vi "Мажор_не_работает_дтектор.vi"() -> ()   [LabVIEW 2017]
panel:
  out "s? t:f":dbl
  out "element":dbl
  out "После ошибки":dbl[](array[numeric])
  out "2-х массив на выходе 3":dbl[][](array[numeric])
  in  "Размер окна":i32=4
  out "см. 1.5":dbl[][](array[numeric])
  out "Декодированное сообщение":dbl[](array[numeric])
  out "Детектированное сообщение":dbl[](array[numeric])
  out "До ошибки":dbl[](array[numeric])
  in  "Кол-во копий":i32=5
  out "Массиве":dbl[](array[numeric])
  in  "Кол-во элементов":i32=16
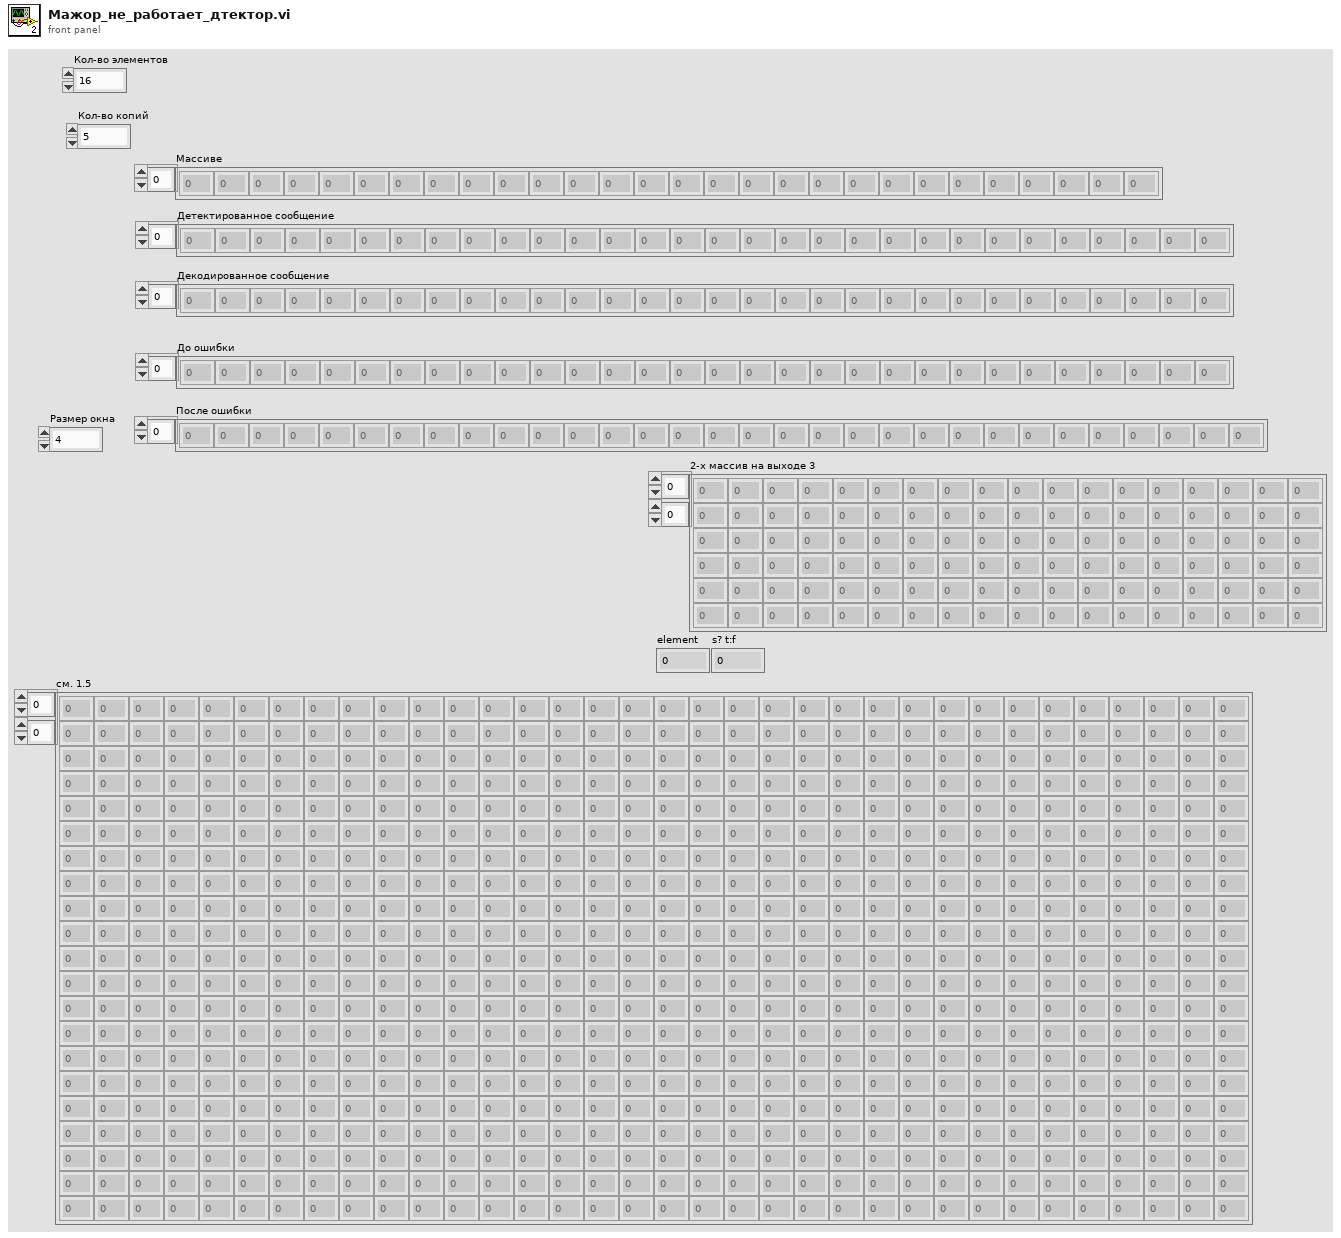
[diagram p1: front panel]
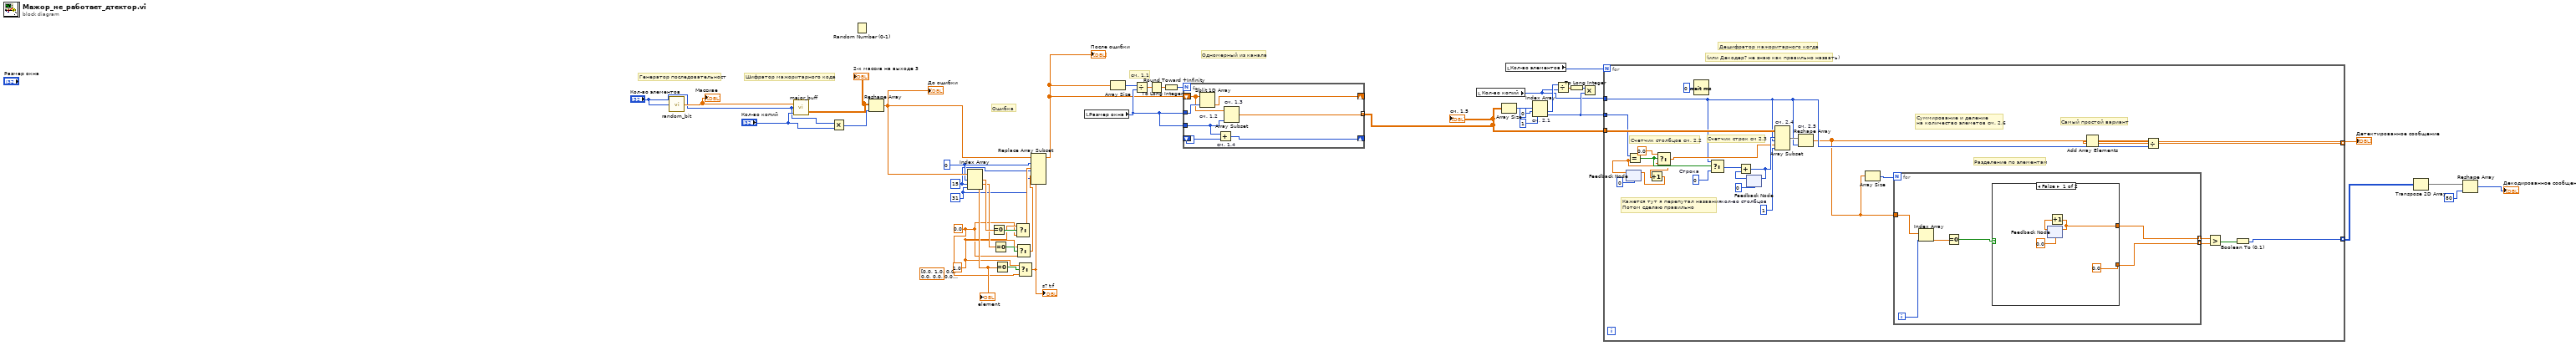
[diagram p0: block diagram]
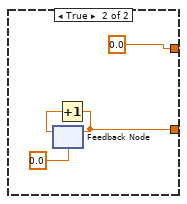
[diagram p2: hidden frame]
diagram:
  (unwired) dbl[] [0.0, 1.0, 0.0, 0.0, 0.0, 0.0, 0.0, 1.0, 1.0, 1.0, 0.0, 1.0, 1.0, 0.0, 0.0, 1.0] ("Декодированное сообщение")
  w12 = 1.0
  w11 = 0.0
  w5 = 31
  w6 = 15
  w7 = 0
  # "Ошибка"
  # "Одномерный из канала"
  # "см. 1.1"
  # "(или Декодер? не знаю как правильно назвать)"
  # "Дешифратор мажоритарного когда"
  # "Шифратор мажоритарного кода"
  # "Генератор последовательност"
  n1 = call "random_bit.vi"("Количество бит"="Кол-во элементов") -> ("Биты на выходе 1"=w41:dbl[])
  "Массиве" <- w41
  n2 = call "major_buff.vi"("Кол-во копий"="Кол-во копий", "Размер окна"="Кол-во элементов", "Биты на выходе 1"=w41) -> ("Подготовленный к отправке мажоритарный код"=w21:dbl[][])  [unwired: 1 out]
  "2-х массив на выходе 3" <- w21
  n3 = Multiply(x="Кол-во элементов", y="Кол-во копий") -> (x*y=w40:i32)
  n4 = Random Number (0-1)() -> ()  [unwired: 1 out]
  n5 = Reshape Array(w21, w40) -> (w19:dbl[])
  "До ошибки" <- w19
  n6 = Index Array(array=w19, index #1=w7, index #2=w6, index #3=w5) -> (element #1=w18:dbl, element #2=w17:dbl, element #3=w16:dbl)
  "element" <- w16
  n7 = Equal To 0?(x=w18) -> (x = 0?=w15:bool)
  n8 = Equal To 0?(x=w17) -> (x = 0?=w14:bool)
  n9 = Equal To 0?(x=w16) -> (x = 0?=w13:bool)
  n10 = Select(t=w12, s=w15, f=w11) -> (s? t:f=w10:dbl)
  n11 = Select(t=w12, s=w14, f=w11) -> (s? t:f=w9:dbl)
  n12 = Select(t=w12, s=w13, f=w11) -> (s? t:f=w8:dbl)
  "s? t:f" <- w8
  n13 = Replace Array Subset(array=w19, new element #1=w10, index #1=w7, new element #2=w9, index #2=w6, new element #3=w8, index #3=w5) -> (w24:dbl[])
  "После ошибки" <- w24
  n14 = local read "Размер окна"() -> (w31:i32)
  n15 = Array Size(array=w24) -> (size(s)=w30:i32)
  n16 = Divide(x=w30, y=w31) -> (x/y=w29:dbl)
  n17 = Round Toward +Infinity(x=w29) -> (ceil(x): smallest int >= x=w28:dbl)
  n18 = To Long Integer(number=w28) -> (32bit integer=w27:i32)
  n19 = for {
    N: w27 -> [_]
    shift-right: [w48] -> _
    shift-left: w24 -> [w46]
    tunnel: w31 -> [w47]
    shift-right: [w44] -> _
    shift-left: _ -> [w43]
    tunnel: w31 -> [w45]
    tunnel: [w42] -> w20 mode=indexing
    n20 = Split 1D Array "см. 1.2"(array=w46, index=w47) -> (second subarray=w48:dbl[])  [unwired: 1 out]
    n21 = Add "см. 1.4"(x=w45, y=w43) -> (x+y=w44:i32)
    n22 = Array Subset "см. 1.3"(array=w46, length=w45) -> (w42:dbl[])  [unwired: 1 in]
  }
  "см. 1.5" <- w20
  n23 = local read "Кол-во копий"() -> (w32:i32)
  n24 = Array Size(array=w20) -> (size(s)=w39:i32[])
  n25 = local read "Кол-во элементов"() -> (w25:i32)
  n26 = Index Array "см. 2.1"(array=w39, index #1=0 ("index"), index #2=1 ("index")) -> (element #1=w36:i32, element #2=w35:i32)
  n27 = Divide(x=w36, y=w32) -> (x/y=w34:dbl)
  n28 = To Long Integer(number=w34) -> (32bit integer=w33:i32)
  n29 = Multiply(x=w33, y=w35) -> ()  [unwired: 1 out]
  n30 = for {
    N: w25 -> [_]
    tunnel: w20 -> [w72]
    tunnel: w35 -> [w64]
    tunnel: w32 -> [w56]
    tunnel: [w55] -> w26 mode=indexing
    tunnel: [w49] -> w4 mode=indexing
    w71 = 1  # кол-во столбцов
    w62 = 0  # Строка
    # "Разделение по элементам"
    # "Самый простой вариант"
    # "Суммирование и деление \nна количество элеметов см. 2.6"
    # "Кажется тут я перепутал названия  \nПотом сделаю правильно"
    # "Счетчик строк см 2.3"
    # "Счетчик столбцов см. 2.2"
    n31 = feedback #1(0) -> (w60:dbl)
    n32 = Equal?(x=w64, y=w60) -> (x = y?=w66:bool)
    n33 = Select(t=0.0, s=w66, f=w60) -> (s? t:f=w59:dbl)
    n34 = Increment(x=w59) -> (x+1=w58:dbl)
    n35 = feedback-in #1(w58) -> ()
    n36 = Wait (ms)(milliseconds to wait=u32 0) -> ()  [unwired: 1 out]
    n37 = Select(t=w56, s=w66, f=w62) -> (s? t:f=w63:i32)
    n38 = feedback #2(0) -> (w65:i32)
    n39 = Add(x=w63, y=w65) -> (x+y=w61:i32)
    n40 = feedback-in #2(w61) -> ()
    n41 = Array Subset "см. 2.4"(array=w72, index (row)=w61, length (row)=w56, index (col)=w59, length (col)=w71) -> (w73:dbl[][])
    n42 = Reshape Array "см. 2.5"(w73, w56) -> (w53:dbl[])
    n43 = Array Size(array=w53) -> (size(s)=w54:i32)
    n44 = for {
      N: w54 -> [_]
      tunnel: w53 -> [w79]
      tunnel: [w75] -> w52 mode=indexing
      tunnel: [w74] -> w51 mode=indexing
      i -> [w78]
      n45 = Index Array(array=w79, index=w78) -> (element=w77:dbl)
      n46 = Equal To 0?(x=w77) -> (x = 0?=w76:bool)
      n47 = case shown="False" w76 {
        tunnel: [0.0 w85] -> w74
        tunnel: [w80 0.0] -> w75
        frame False {
          n48 = feedback #3(0.0) -> (w81:dbl)
          n49 = Increment(x=w81) -> (x+1=w80:dbl)
          n50 = feedback-in #3(w80) -> ()
        }
        frame True {
          n51 = feedback #4(0.0) -> (w86:dbl)
          n52 = Increment(x=w86) -> (x+1=w85:dbl)
          n53 = feedback-in #4(w85) -> ()
        }
      }
    }
    n54 = Add Array Elements(numeric array=w53) -> (sum=w57:dbl)
    n55 = Divide(x=w57, y=w56) -> (x/y=w55:dbl)
    n56 = Greater?(x=w52, y=w51) -> (0:w50:bool[])
    n57 = Boolean To (0,1)(Boolean=w50) -> (0, 1=w49:i16[])
  }
  "Детектированное сообщение" <- w26
  n58 = Transpose 2D Array(2D array=w4) -> (transposed array=w2:i16[][])
  n59 = Reshape Array(w2, 80) -> (→"Декодированное сообщение":i16[])
